vi "Handle Exit.vi"(8 "error in (no error)":errorcluster, 10 "Stop Argument":T1, 11 "Vi Ref":refnum<vi>) -> (0 "error out":errorcluster)   [LabVIEW 2014, in "Chart Module.lvlib"]
uses:
  Chart Module.lvlib
  Stop Argument--cluster.ctl
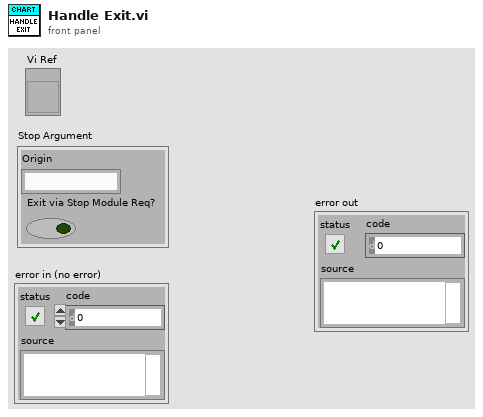
[diagram p1: front panel]
types:
  T1 = typedef "Chart Module.lvlib/Stop Argument--cluster.ctl" = cluster{"Origin":string, "Exit via Stop Module Req?":bool}
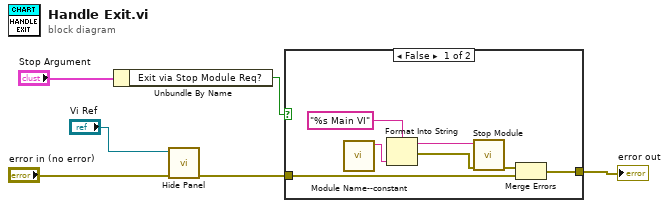
[diagram p0: block diagram]
diagram:
  n1 = Unbundle By Name("Stop Argument") -> ("Exit via Stop Module Req?"=w4:bool)
  n2 = call "Hide Panel.vi"("error in (no error)"="error in (no error)", "Vi Ref"="Vi Ref") -> ("error out"=w2:errorcluster)  [unwired: 9 in]
  n3 = case shown="False" w4 {
    tunnel: w2 -> [w8 w14]
    tunnel: [w7 w14] -> w3
    frame False {
      n4 = call "Module Name--constant.vi"() -> ("Module Name"=w12:string)  [unwired: 11 in]
      n5 = Format Into String(format string="%s Main VI", w12) -> (resulting string=w11:string, error out=w10:errorcluster)  [unwired: 2 in]
      n6 = call "Stop Module.vi"("error in (no error)"=w10, "Origin"=w11) -> ("error out"=w9:errorcluster)  [unwired: 9 in]
      n7 = Merge Errors(w9, w8) -> (w7:errorcluster)
    }
    frame True {
      # "no need to call stop module again"
    }
  }
  "error out" <- w3
